vi "conditional index even number array.vi"() -> ()   [LabVIEW 2023]
panel:
  out "else do nothing":i32[](array[numeric])
  in  "Array 2":i32[](array[numeric])
  out "conditional index":dbl[](array[numeric])
  in  "array":dbl[](array[numeric])
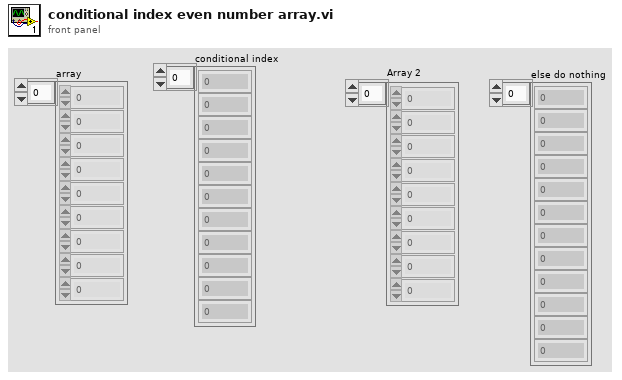
[diagram p1: front panel]
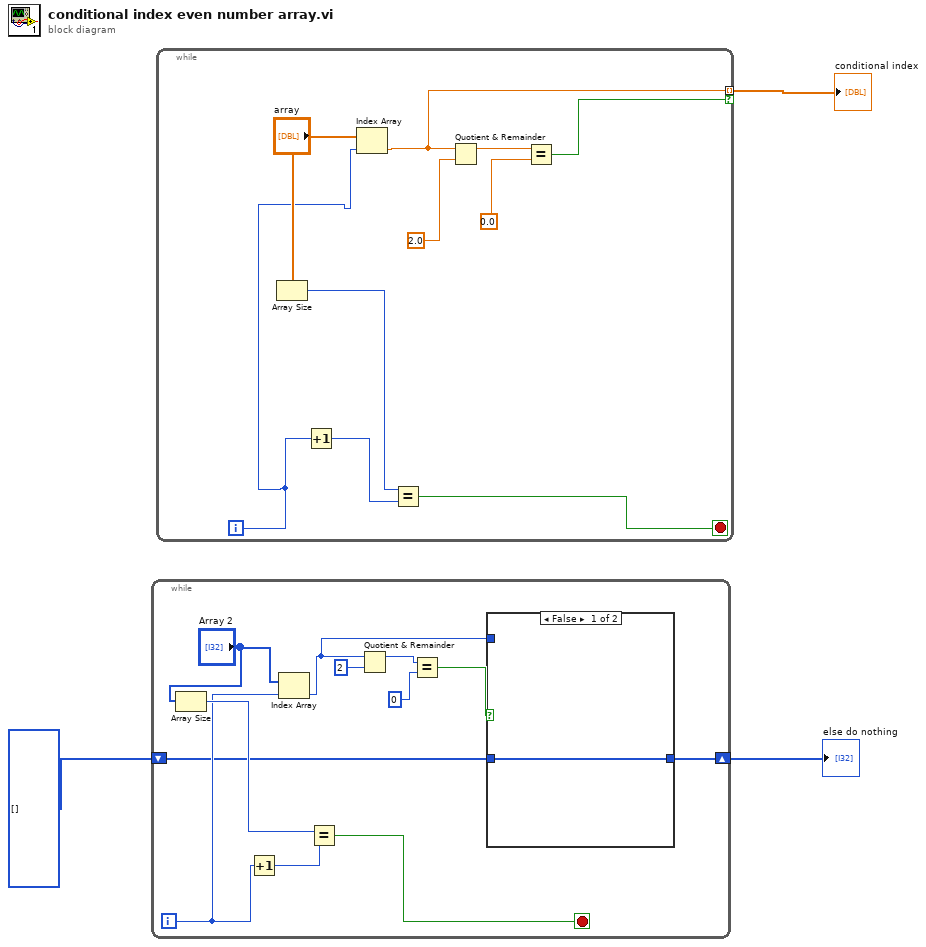
[diagram p0: block diagram]
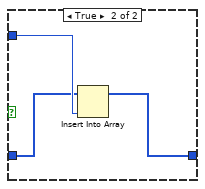
[diagram p2: hidden frame]
diagram:
  n1 = while {
    shift-right: [w4] -> w2
    shift-left: i32[] [] -> [w6]
    i -> [w11]
    stop <- w12 stop-if-true
    n2 = Array Size(array="Array 2") -> (size(s)=w14:i32)
    n3 = Increment(x=w11) -> (x+1=w13:i32)
    n4 = Index Array(array="Array 2", index=w11) -> (element=w5:i32)
    n5 = Equal?(x=w14, y=w13) -> (x = y?=w12:bool)
    n6 = Quotient & Remainder(x=w5, y=2) -> (x-y*floor(x/y)=w9:i32)  [unwired: 1 out]
    n7 = Equal?(x=w9, y=0) -> (x = y?=w7:bool)
    n8 = case shown="False" w7 {
      tunnel: w6 -> [w16 w18]
      tunnel: w5 -> [_ w19]
      tunnel: [w16 w17] -> w4
      frame False {
      }
      frame True {
        n9 = Insert Into Array(array=w18, new element=w19) -> (w17:i32[])  [unwired: 1 in]
      }
    }
  }
  "else do nothing" <- w2
  n10 = while {
    tunnel: [w21] -> w3 mode=indexing if=w20
    i -> [w25]
    stop <- w26 stop-if-true
    n11 = Array Size(array="array") -> (size(s)=w27:i32)
    n12 = Increment(x=w25) -> (x+1=w28:i32)
    n13 = Index Array "Index Array"(array="array", index=w25) -> (element=w21:dbl)
    n14 = Equal?(x=w27, y=w28) -> (x = y?=w26:bool)
    n15 = Quotient & Remainder(x=w21, y=2.0) -> (x-y*floor(x/y)=w23:dbl)  [unwired: 1 out]
    n16 = Equal?(x=w23, y=0.0) -> (x = y?=w20:bool)
  }
  "conditional index" <- w3
